vi "ReadRouterState.vi"(8 "error in (no error)":errorcluster, 11 "AdsNET in":refnum<class "AdsNET.lvclass">) -> (0 "error out":errorcluster, 2 "RouterState":i32(ring) items=["Stop", "Start", "Removed"], 3 "AdsNET out":refnum<class "AdsNET.lvclass">)   [LabVIEW 2016, in "TCatAdsNet.lvlib" / "AdsNET.lvclass"]
doc: "Gets the current state of the local AMS Router"
uses:
  AdsNET.lvclass
  AdsNET.lvclass/AdsNET.ctl
  C:/Users/Maurizio/Projects/sentiero-beckoff/DLL/TwinCAT.Ads.dll
  sentiero-beckoff/DLL/TwinCAT.Ads.dll
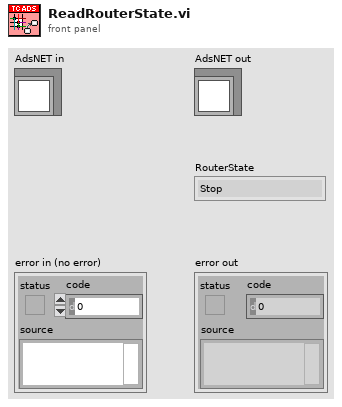
[diagram p1: front panel]
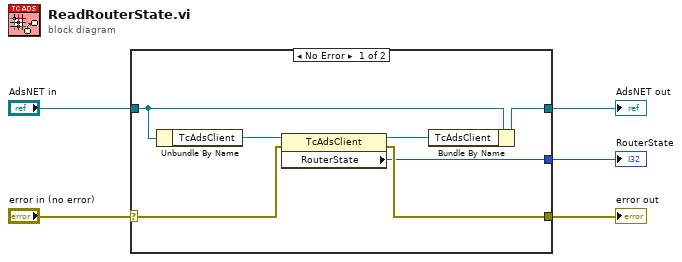
[diagram p0: block diagram]
diagram:
  n1 = case shown="No Error" "error in (no error)" {
    selector: "error in (no error)" -> [w8 w14]
    tunnel: [w7 w14] -> w4
    tunnel: [w10 w13] -> w2
    tunnel: "AdsNET in" -> [w12 w13]
    tunnel: [w6 _] -> w1
    frame No Error {
      n2 = Unbundle By Name(w12) -> ("TcAdsClient"=w11:refnum<k24>)
      n3 = property class="TcAdsClient"(reference=w11, error in=w8) -> (reference out=w9:refnum<k24>, error out=w7:errorcluster, "RouterState"=w6:i32)
      n4 = Bundle By Name(cluster=w12, "TcAdsClient"=w9) -> (w10:refnum<class "AdsNET.lvclass">)
    }
    frame Error {
    }
  }
  "error out" <- w4
  "AdsNET out" <- w2
  "RouterState" <- w1
